vi "Relay_Load_and_PV_v02 (9039).vi"() -> ()   [LabVIEW 2015]
uses:
  subVIs/Load case typedef.ctl
  <vilib>/Modbus/slave/Create Slave Instance (TCP).vi
  <vilib>/FPGAPlugInAG/cRIO-9039/niLvFpga_Open_cRIO-9039.vi
  <vilib>/rvi/interface/common/dynamic/niFpgaDynamicAddResources.vi
  <vilib>/Utility/error.llb/Error Cluster From Error Code.vi
  <vilib>/rvi/errors/niLvFpgaAdjustHostInterfaceError.vi
  <vilib>/FPGAPlugInAG/Dynamic/niLvFpga_Close_Dynamic.vi
  <vilib>/rvi/interface/nirviOpenFPGA/nirviOpenFPGA.xnode
  FPGA Bitfiles/RTDSLoadControl_FPGATarget_9309.lvbitx
  <vilib>/rvi/interface/nirviReadWriteControl/nirviReadWriteControl.xnode
  <vilib>/rvi/interface/nirviCloseFPGA/nirviCloseFPGA.xnode
  <vilib>/Modbus/slave/Modbus Slave.lvclass
  2015 SP1 Support Files/Project Dependencies/Common/Modbus Data Conversion.llb/Modbus Data Conversion.lvlib
  NiFpgaLv.dll
  <vilib>/rvi/interface/Simulation/niFpgaSimulationCallBeginRW.vi
panel:
  out "error out":errorcluster
  out "Load array":sgl[](array[numeric])
  out "PV array":sgl[](array[numeric])
  out "Loop dT (Ticks)":u32
  in  "Loop Rate (Ticks)":u32=1000
  out "Activate Command PV":bool
  out "Deactivate Command PV":bool
  out "Activation Status PV":bool
  out "Deactivation Status PV":bool=TRUE
  out "TCP \nConnection Count PV":u32
  out "comm stopped PV":bool
  in  "Input register\naddresses PV":T1={"Ia"=30030, "Ib"=30040, "Ic"=30050, "Va"=30130, "Vb"=30140, "Vc"=30150, "Pa"=30230, "Pb"=30240, "Pc"=30250, "Qa"=30330, "Qb"=30340, "Qc"=30350}
  in  "Input \nregister values PV":T2
  out "Modbus Data PV":T3
  out "S Total PV":dbl
  out "P Total PV":dbl
  out "Q Total PV":dbl
  out "Q Total":dbl
  out "P Total":dbl
  out "S Total":dbl
  out "Modbus Data":T3
  in  "Input \nregister values":T3
  out "comm stopped":bool
  out "Activate Command":bool
  out "Deactivate Command":bool
  out "Activation Status":bool
  out "Deactivation Status":bool=TRUE
  out "TCP \nConnection Count":u32
  in  "Input register\naddresses":T1={"Ia"=30030, "Ib"=30040, "Ic"=30050, "Va"=30130, "Vb"=30140, "Vc"=30150, "Pa"=30230, "Pb"=30240, "Pc"=30250, "Qa"=30330, "Qb"=30340, "Qc"=30350}
  in  "stop":bool
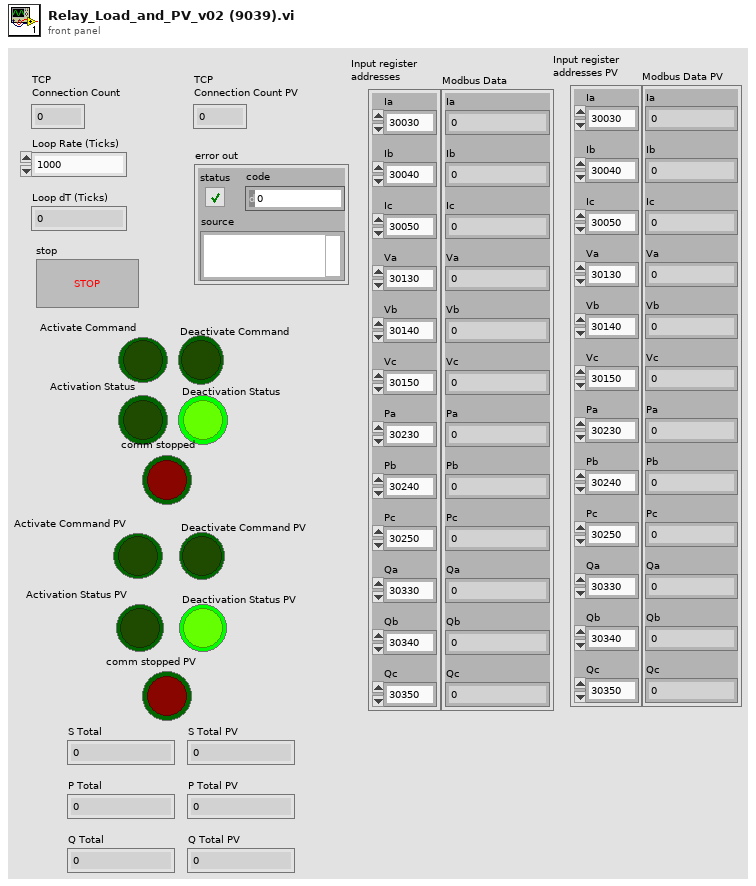
[diagram p1: front panel]
types:
  T1 = cluster{"Ia":u16, "Ib":u16, "Ic":u16, "Va":u16, "Vb":u16, "Vc":u16, "Pa":u16, "Pb":u16, "Pc":u16, "Qa":u16, "Qb":u16, "Qc":u16}
  T2 = cluster{"Ia PV":dbl, "Ib PV":dbl, "Ic PV":dbl, "Va PV":dbl, "Vb PV":dbl, "Vc PV":dbl, "Pa PV":dbl, "Pb PV":dbl, "Pc PV":dbl, "Qa PV":dbl, "Qb PV":dbl, "Qc PV":dbl}
  T3 = cluster{"Ia":dbl, "Ib":dbl, "Ic":dbl, "Va":dbl, "Vb":dbl, "Vc":dbl, "Pa":dbl, "Pb":dbl, "Pc":dbl, "Qa":dbl, "Qb":dbl, "Qc":dbl}
  T4 = typedef "Load case typedef.ctl" = enum16{"Commisioning", "Activation", "Deactivation"}
  T5 = cluster{dbl, dbl, dbl, dbl, dbl, dbl, dbl, dbl, dbl, dbl, dbl, dbl}
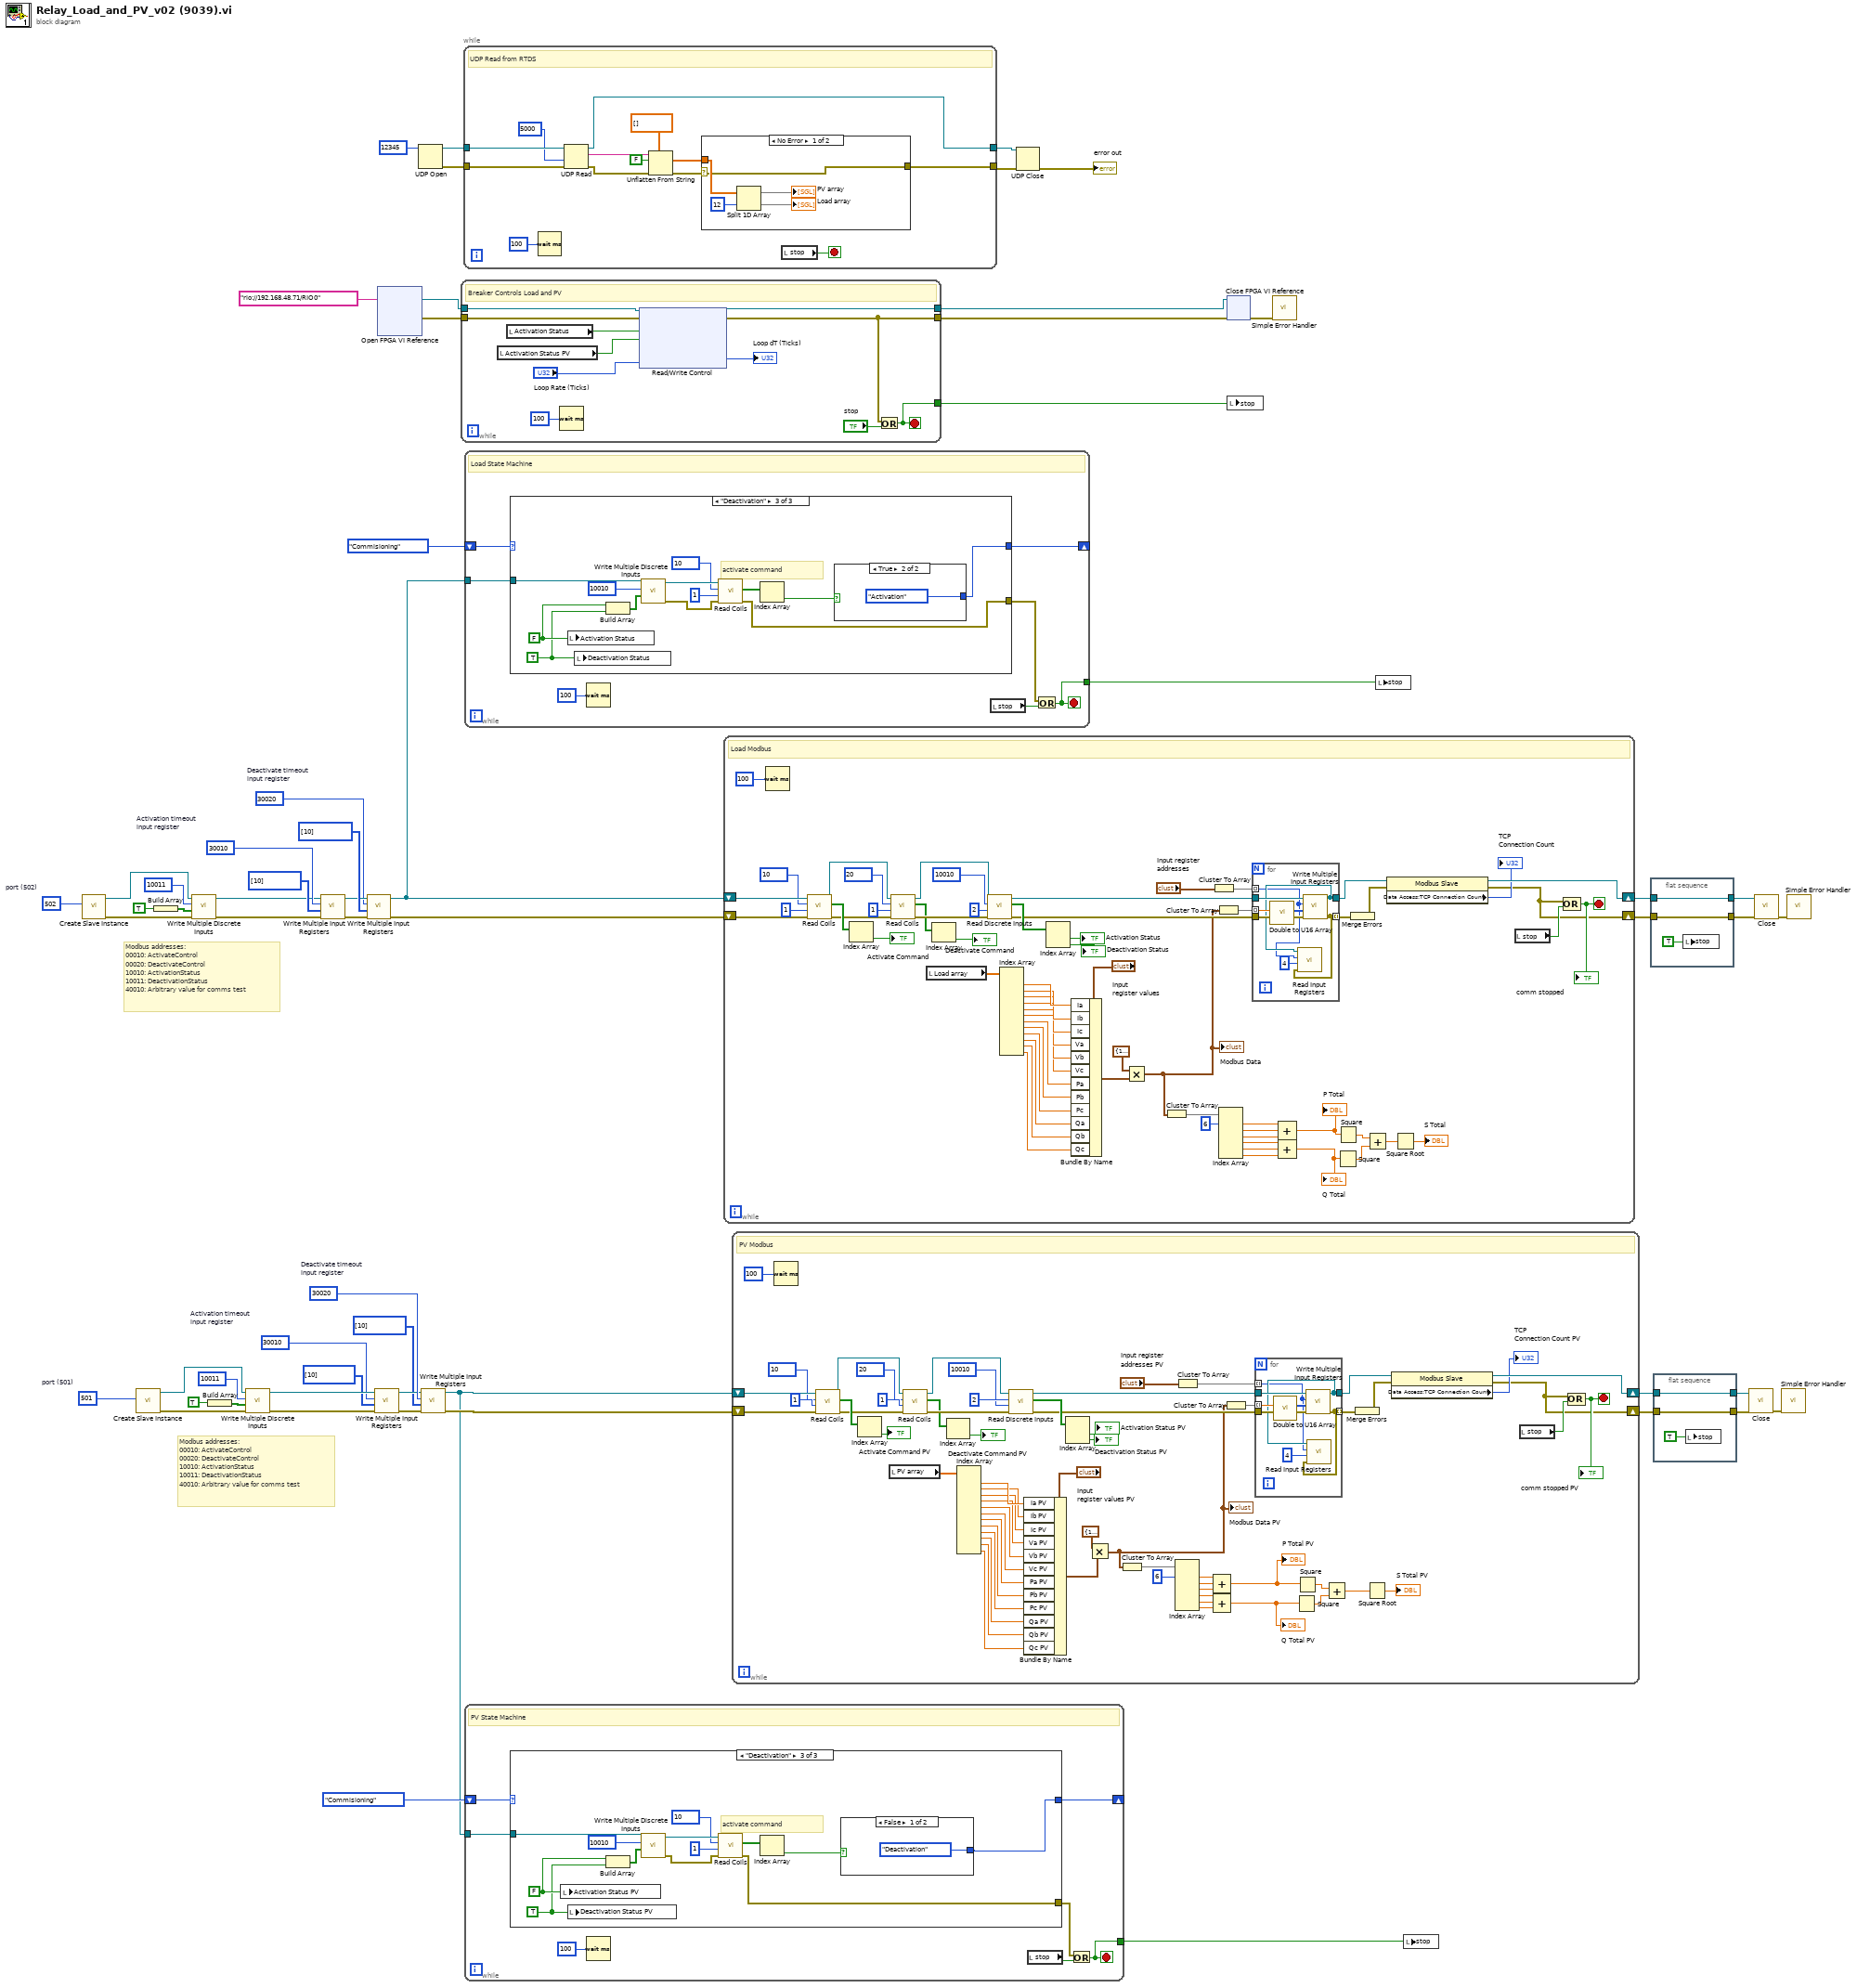
[diagram p0: block diagram]
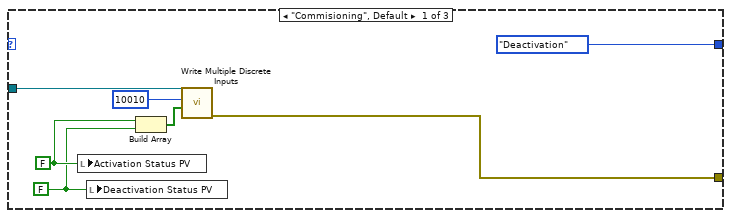
[diagram p3: hidden frame]
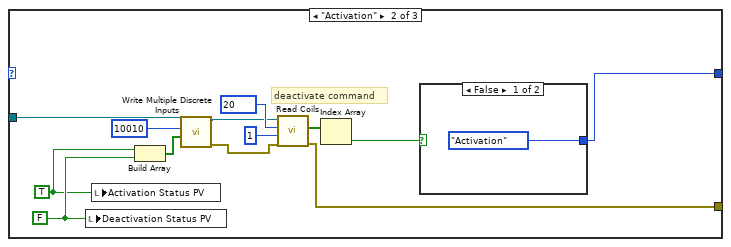
[diagram p4: hidden frame]
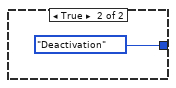
[diagram p5: hidden frame]
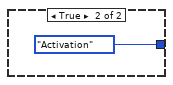
[diagram p6: hidden frame]
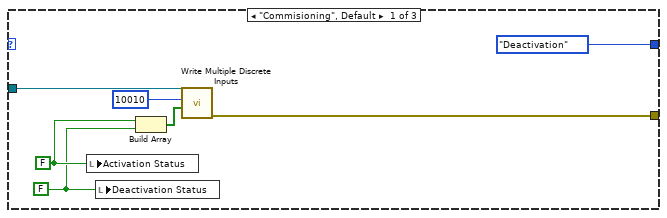
[diagram p7: hidden frame]
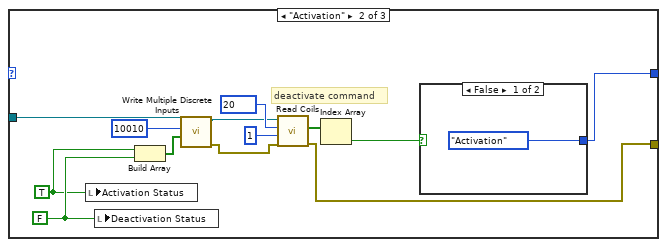
[diagram p8: hidden frame]
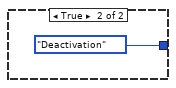
[diagram p9: hidden frame]
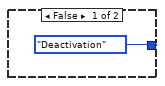
[diagram p10: hidden frame]
diagram:
  w28 = u16 501  # port (501)
  w32 = u16 30020  # Deactivate timeout input register
  w34 = u16 30010  # Activation timeout input register
  w53 = u16 502  # port (502)
  w45 = u16 30020  # Deactivate timeout input register
  w43 = u16 30010  # Activation timeout input register
  # "Modbus addresses:\n00010: ActivateControl\n00020: DeactivateControl\n10010: ActivationStatus\n10011: DeactivationStatus\n40010: Arbitrary value for comms test"
  # "Modbus addresses:\n00010: ActivateControl\n00020: DeactivateControl\n10010: ActivationStatus\n10011: DeactivationStatus\n40010: Arbitrary value for comms test"
  n1 = call-poly <vilib>:"Create Slave Instance.vi"("port (502)"=w53) -> ("error out"=w57:errorcluster, "TCP slave instance"=w58:refnum<class "Modbus Slave.lvclass">)  [unwired: 9 in]
  n2 = call-poly <vilib>:"Create Slave Instance.vi"("port (502)"=w28) -> ("error out"=w24:errorcluster, "TCP slave instance"=w23:refnum<class "Modbus Slave.lvclass">)  [unwired: 9 in]
  n3 = Build Array(TRUE ("Activate 2")) -> (w54:bool[])
  n4 = call-dynamic "Write Multiple Discrete Inputs.vi"("error in (no error)"=w57, "discrete input values"=w54, "starting address"=u16 10011, "Modbus slave in"=w58) -> ("error out"=w41:errorcluster, "Modbus slave out"=w42:refnum<class "Modbus Slave.lvclass">)  [unwired: 6 in]
  n5 = Build Array(TRUE ("Activate 2")) -> (w27:bool[])
  n6 = call-dynamic "Write Multiple Discrete Inputs.vi"("error in (no error)"=w24, "discrete input values"=w27, "starting address"=u16 10011, "Modbus slave in"=w23) -> ("error out"=w36:errorcluster, "Modbus slave out"=w35:refnum<class "Modbus Slave.lvclass">)  [unwired: 6 in]
  n7 = call-dynamic "Write Multiple Input Registers.vi"("error in (no error)"=w41, "input register values"=u16[] [10], "starting address"=w43, "Modbus slave in"=w42) -> ("error out"=w47:errorcluster, "Modbus slave out"=w46:refnum<class "Modbus Slave.lvclass">)  [unwired: 6 in]
  n8 = call-dynamic "Write Multiple Input Registers.vi"("error in (no error)"=w47, "input register values"=u16[] [10], "starting address"=w45, "Modbus slave in"=w46) -> ("error out"=w39:errorcluster, "Modbus slave out"=w40:refnum<class "Modbus Slave.lvclass">)  [unwired: 6 in]
  n9 = call-dynamic "Write Multiple Input Registers.vi"("error in (no error)"=w36, "input register values"=u16[] [10], "starting address"=w34, "Modbus slave in"=w35) -> ("error out"=w30:errorcluster, "Modbus slave out"=w31:refnum<class "Modbus Slave.lvclass">)  [unwired: 6 in]
  n10 = xnode "Open FPGA VI Reference"("resource name"=tag "rio://192.168.48.71/RIO0") -> ("FPGA VI Reference Out"=w51:refnum<k20>, "error out"=w50:errorcluster)  [unwired: 1 in]
  n11 = UDP Open(11:u16 12345 ("port")) -> (port=w4:refnum<k16>, 0:w3:errorcluster)  [unwired: 4 in, 1 out]
  n12 = call-dynamic "Write Multiple Input Registers.vi"("error in (no error)"=w30, "input register values"=u16[] [10], "starting address"=w32, "Modbus slave in"=w31) -> ("error out"=w22:errorcluster, "Modbus slave out"=w19:refnum<class "Modbus Slave.lvclass">)  [unwired: 6 in]
  n13 = while {
    tunnel: [w70] -> w52
    tunnel: w51 -> [w69]
    tunnel: w50 -> [w68]
    tunnel: [w61] -> w49
    tunnel: [w60] -> w9
    stop <- w60 stop-if-true
    # "Breaker Controls Load and PV"
    n14 = local read "Activation Status PV"() -> (w65:bool)
    n15 = local read "Activation Status"() -> (w67:bool)
    n16 = Wait (ms)(milliseconds to wait=u32 100) -> ()  [unwired: 1 out]
    n17 = xnode "Read/Write Control"("FPGA VI Reference In"=w69, "error in"=w68, "Load Relay closed"=w67, "PV Relay closed"=w65, "Loop Rate (Ticks)"="Loop Rate (Ticks)") -> ("FPGA VI Reference Out"=w70:refnum<k20>, "error out"=w61:errorcluster, "Loop dT (Ticks)"=→"Loop dT (Ticks)":u32)
    n18 = Or(x=w61, y="stop") -> (x .or. y?=w60:bool)
  }
  n19 = while {
    tunnel: [w75] -> w2
    tunnel: [w74] -> w5
    tunnel: w4 -> [w73]
    tunnel: w3 -> [w72]
    stop <- w83 stop-if-true
    # "UDP Read from RTDS"
    n20 = Wait (ms)(milliseconds to wait=u32 100) -> ()  [unwired: 1 out]
    n21 = UDP Read(connection ID=w73, timeout ms (25000)=5000, 8:w72) -> (data out=w82:string, error out=w81:errorcluster, 3:w74:refnum<k16>)  [unwired: 1 in, 2 out]
    n22 = Unflatten From String(type=sgl[] [], binary string=w82, data includes array or string size? (T)=FALSE, error in (no error)=w81) -> (value=w78:sgl[], error out=w77:errorcluster)  [unwired: 1 in, 1 out]
    n23 = case shown="No Error" w77 {
      selector: w77 -> [w84 w89]
      tunnel: w78 -> [w88 _]
      tunnel: [w84 w89] -> w75
      frame No Error {
        n24 = Split 1D Array(array=w88, index=12 ("length")) -> (first subarray=→"PV array":sgl[], second subarray=→"Load array":sgl[])
      }
      frame Error {
      }
    }
    n25 = local read "stop"() -> (w83:bool)
  }
  n26 = while {
    tunnel: w40 -> [w94]
    shift-right: [w93] -> _
    shift-left: Load_case_typedef."Commisioning" ("Load enum") -> [w95]
    tunnel: [w90] -> w8
    stop <- w90 stop-if-true
    # "Load State Machine"
    n27 = case shown="\"Deactivation\"" w95 {
      tunnel: w94 -> [w101 w112 w127]
      tunnel: [Load_case_typedef."Deactivation" ("Load enum") w106 w121] -> w93
      tunnel: [w97 w104 w119] -> w92
      frame "Commisioning", Default {
        w99 = FALSE ("Deactivation Status")
        w100 = FALSE ("Activation Status")
        n28 = local write "Activation Status"(w100) -> ()
        n29 = local write "Deactivation Status"(w99) -> ()
        n30 = Build Array(w100, w99) -> (w103:bool[])
        n31 = call-dynamic "Write Multiple Discrete Inputs.vi"("discrete input values"=w103, "starting address"=u16 10010, "Modbus slave in"=w101) -> ("error out"=w97:errorcluster)  [unwired: 7 in, 1 out]
      }
      frame "Activation" {
        w116 = FALSE ("Deactivation Status")
        w115 = TRUE ("Activation Status")
        # "deactivate command"
        n32 = local write "Activation Status"(w115) -> ()
        n33 = local write "Deactivation Status"(w116) -> ()
        n34 = Build Array(w115, w116) -> (w113:bool[])
        n35 = call-dynamic "Write Multiple Discrete Inputs.vi"("discrete input values"=w113, "starting address"=u16 10010, "Modbus slave in"=w112) -> ("error out"=w105:errorcluster, "Modbus slave out"=w108:refnum<class "Modbus Slave.lvclass">)  [unwired: 7 in]
        n36 = call-dynamic "Read Coils.vi"("error in (no error)"=w105, "number of coils"=u16 1, "starting address"=u16 20, "Modbus slave in"=w108) -> ("error out"=w104:errorcluster, "coil values"=w109:bool[])  [unwired: 5 in, 1 out]
        n37 = Index Array(array=w109) -> (element=w107:bool)  [unwired: 1 in]
        n38 = case shown="False" w107 {
          tunnel: [Load_case_typedef."Activation" ("Load enum") Load_case_typedef."Deactivation" ("Load enum")] -> w106
          frame False {
          }
          frame True {
          }
        }
      }
      frame "Deactivation" {
        w128 = TRUE ("Deactivation Status")
        w129 = FALSE ("Activation Status")
        # "activate command"
        n39 = local write "Activation Status"(w129) -> ()
        n40 = local write "Deactivation Status"(w128) -> ()
        n41 = Build Array(w129, w128) -> (w131:bool[])
        n42 = call-dynamic "Write Multiple Discrete Inputs.vi"("discrete input values"=w131, "starting address"=u16 10010, "Modbus slave in"=w127) -> ("error out"=w120:errorcluster, "Modbus slave out"=w126:refnum<class "Modbus Slave.lvclass">)  [unwired: 7 in]
        n43 = call-dynamic "Read Coils.vi"("error in (no error)"=w120, "number of coils"=u16 1, "starting address"=u16 10, "Modbus slave in"=w126) -> ("error out"=w119:errorcluster, "coil values"=w123:bool[])  [unwired: 5 in, 1 out]
        n44 = Index Array(array=w123) -> (element=w122:bool)  [unwired: 1 in]
        n45 = case shown="True" w122 {
          tunnel: [Load_case_typedef."Deactivation" ("Load enum") Load_case_typedef."Activation" ("Load enum")] -> w121
          frame False {
          }
          frame True {
          }
        }
      }
    }
    n46 = Wait (ms)(milliseconds to wait=u32 100) -> ()  [unwired: 1 out]
    n47 = local read "stop"() -> (w91:bool)
    n48 = Or(x=w92, y=w91) -> (x .or. y?=w90:bool)
  }
  n49 = while {
    tunnel: w19 -> [w138]
    shift-right: [w137] -> _
    shift-left: Load_case_typedef."Commisioning" ("Load enum") -> [w139]
    tunnel: [w134] -> w7
    stop <- w134 stop-if-true
    # "PV State Machine"
    n50 = case shown="\"Deactivation\"" w139 {
      tunnel: w138 -> [w145 w156 w171]
      tunnel: [Load_case_typedef."Deactivation" ("Load enum") w150 w165] -> w137
      tunnel: [w141 w148 w163] -> w135
      frame "Commisioning", Default {
        w143 = FALSE ("Deactivation Status")
        w144 = FALSE ("Activation Status")
        n51 = local write "Activation Status PV"(w144) -> ()
        n52 = local write "Deactivation Status PV"(w143) -> ()
        n53 = Build Array(w144, w143) -> (w147:bool[])
        n54 = call-dynamic "Write Multiple Discrete Inputs.vi"("discrete input values"=w147, "starting address"=u16 10010, "Modbus slave in"=w145) -> ("error out"=w141:errorcluster)  [unwired: 7 in, 1 out]
      }
      frame "Activation" {
        w160 = FALSE ("Deactivation Status")
        w159 = TRUE ("Activation Status")
        # "deactivate command"
        n55 = local write "Deactivation Status PV"(w160) -> ()
        n56 = local write "Activation Status PV"(w159) -> ()
        n57 = Build Array(w159, w160) -> (w157:bool[])
        n58 = call-dynamic "Write Multiple Discrete Inputs.vi"("discrete input values"=w157, "starting address"=u16 10010, "Modbus slave in"=w156) -> ("error out"=w149:errorcluster, "Modbus slave out"=w152:refnum<class "Modbus Slave.lvclass">)  [unwired: 7 in]
        n59 = call-dynamic "Read Coils.vi"("error in (no error)"=w149, "number of coils"=u16 1, "starting address"=u16 20, "Modbus slave in"=w152) -> ("error out"=w148:errorcluster, "coil values"=w153:bool[])  [unwired: 5 in, 1 out]
        n60 = Index Array(array=w153) -> (element=w151:bool)  [unwired: 1 in]
        n61 = case shown="False" w151 {
          tunnel: [Load_case_typedef."Activation" ("Load enum") Load_case_typedef."Deactivation" ("Load enum")] -> w150
          frame False {
          }
          frame True {
          }
        }
      }
      frame "Deactivation" {
        w172 = TRUE ("Deactivation Status")
        w173 = FALSE ("Activation Status")
        # "activate command"
        n62 = local write "Activation Status PV"(w173) -> ()
        n63 = local write "Deactivation Status PV"(w172) -> ()
        n64 = Build Array(w173, w172) -> (w175:bool[])
        n65 = call-dynamic "Write Multiple Discrete Inputs.vi"("discrete input values"=w175, "starting address"=u16 10010, "Modbus slave in"=w171) -> ("error out"=w164:errorcluster, "Modbus slave out"=w170:refnum<class "Modbus Slave.lvclass">)  [unwired: 7 in]
        n66 = call-dynamic "Read Coils.vi"("error in (no error)"=w164, "number of coils"=u16 1, "starting address"=u16 10, "Modbus slave in"=w170) -> ("error out"=w163:errorcluster, "coil values"=w167:bool[])  [unwired: 5 in, 1 out]
        n67 = Index Array(array=w167) -> (element=w166:bool)  [unwired: 1 in]
        n68 = case shown="False" w166 {
          tunnel: [Load_case_typedef."Deactivation" ("Load enum") Load_case_typedef."Activation" ("Load enum")] -> w165
          frame False {
          }
          frame True {
          }
        }
      }
    }
    n69 = Wait (ms)(milliseconds to wait=u32 100) -> ()  [unwired: 1 out]
    n70 = local read "stop"() -> (w136:bool)
    n71 = Or(x=w135, y=w136) -> (x .or. y?=w134:bool)
  }
  n72 = while {
    shift-right: [w221] -> w16
    shift-left: w40 -> [w237]
    shift-right: [w178] -> w17
    shift-left: w39 -> [w236]
    stop <- w240 stop-if-true
    # "Load Modbus"
    n73 = Wait (ms)(milliseconds to wait=u32 100) -> ()  [unwired: 1 out]
    n74 = call-dynamic "Read Coils.vi"("error in (no error)"=w236, "number of coils"=u16 1, "starting address"=u16 10, "Modbus slave in"=w237) -> ("error out"=w229:errorcluster, "coil values"=w241:bool[], "Modbus slave out"=w226:refnum<class "Modbus Slave.lvclass">)  [unwired: 5 in]
    n75 = Index Array(array=w241) -> (element=→"Activate Command":bool)  [unwired: 1 in]
    n76 = call-dynamic "Read Coils.vi"("error in (no error)"=w229, "number of coils"=u16 1, "starting address"=u16 20, "Modbus slave in"=w226) -> ("error out"=w228:errorcluster, "coil values"=w223:bool[], "Modbus slave out"=w227:refnum<class "Modbus Slave.lvclass">)  [unwired: 5 in]
    n77 = local read "Load array"() -> (w194:sgl[])
    n78 = Index Array(array=w223) -> (element=→"Deactivate Command":bool)  [unwired: 1 in]
    n79 = call-dynamic "Read Discrete Inputs.vi"("error in (no error)"=w228, "number of discrete inputs"=u16 2 ("number of coils"), "starting address"=u16 10010 ("address"), "Modbus slave in"=w227) -> ("error out"=w218:errorcluster, "discrete input values"=w234:bool[], "Modbus slave out"=w219:refnum<class "Modbus Slave.lvclass">)  [unwired: 5 in]
    n80 = Index Array(array=w194) -> (element #1=w193:sgl, element #2=w192:sgl, element #3=w191:sgl, element #4=w190:sgl, element #5=w189:sgl, element #6=w188:sgl, element #7=w187:sgl, element #8=w186:sgl, element #9=w185:sgl, element #10=w184:sgl, element #11=w183:sgl, element #12=w182:sgl)  [unwired: 12 in]
    n81 = Index Array(array=w234) -> (element #1=→"Activation Status":bool, element #2=→"Deactivation Status":bool)  [unwired: 2 in]
    n82 = Bundle By Name(cluster="Input \nregister values", "Ia"=w193, "Ib"=w192, "Ic"=w191, "Va"=w190, "Vb"=w189, "Vc"=w188, "Pa"=w187, "Pb"=w186, "Pc"=w185, "Qa"=w184, "Qb"=w183, "Qc"=w182) -> (w215:T3)
    n83 = Multiply(x=T3 {"Ia"=1000.0, "Ib"=1000.0, "Ic"=1000.0, "Va"=1732.0, "Vb"=1732.0, "Vc"=1732.0, "Pa"=1000000.0, "Pb"=1000000.0, "Pc"=1000000.0, "Qa"=1000000.0, "Qb"=1000000.0, "Qc"=1000000.0}, y=w215) -> (x*y=w180:T3)
    "Modbus Data" <- w180
    n84 = Cluster To Array(cluster=w180) -> (array=w181:dbl[])
    n85 = Cluster To Array(cluster="Input register\naddresses") -> (array=w206:u16[])
    n86 = Cluster To Array(cluster=w180) -> (array=w205:dbl[])
    n87 = Index Array(array=w181, index #1=6 ("index")) -> (element #1=w200:dbl, element #2=w199:dbl, element #3=w198:dbl, element #4=w197:dbl, element #5=w195:dbl, element #6=w196:dbl)  [unwired: 5 in]
    n88 = for {
      tunnel: w219 -> [w249]
      tunnel: w218 -> [w248]
      tunnel: [w245] -> w204
      tunnel: [w242] -> w208 mode=indexing
      tunnel: w206 -> [w244] mode=indexing
      tunnel: w205 -> [w246] mode=indexing
      n89 = call "Double to U16 Array.vi"("Double"=w246) -> ("U16 Array"=w247:u16[])  [unwired: 10 in]
      n90 = call-dynamic "Write Multiple Input Registers.vi"("error in (no error)"=w248, "input register values"=w247, "starting address"=w244, "Modbus slave in"=w249) -> ("error out"=w242:errorcluster, "Modbus slave out"=w245:refnum<class "Modbus Slave.lvclass">)  [unwired: 6 in]
      n91 = call-dynamic "Read Input Registers.vi"("error in (no error)"=w242, "number of input registers"=u16 4 ("number of coils"), "starting address"=w244, "Modbus slave in"=w245) -> ()  [unwired: 5 in, 3 out]
    }
    n92 = Compound Arithmetic op=ADD(w200, w199, w198) -> (w201:dbl)
    "P Total" <- w201
    n93 = Compound Arithmetic op=ADD(w197, w195, w196) -> (w202:dbl)
    "Q Total" <- w202
    n94 = Square(x=w202) -> (x^2=w212:dbl)
    n95 = Square(x=w201) -> (x^2=w213:dbl)
    n96 = Merge Errors(w208) -> (w179:errorcluster)
    n97 = Add(x=w213, y=w212) -> (x+y=w211:dbl)
    n98 = property class="Modbus Slave"(reference=w204, error in=w179) -> (reference out=w221:refnum<class "Modbus Slave.lvclass">, error out=w178:errorcluster, "Data Access:TCP Connection Count"=→"TCP \nConnection Count":u32)
    n99 = Square Root(x=w211) -> (sqrt(x)=→"S Total":dbl)
    n100 = local read "stop"() -> (w214:bool)
    n101 = Compound Arithmetic op=OR(w178, w214) -> (w240:bool)
    "comm stopped" <- w240
  }
  n102 = while {
    shift-right: [w293] -> w13
    shift-left: w19 -> [w309]
    shift-right: [w250] -> w12
    shift-left: w22 -> [w308]
    stop <- w312 stop-if-true
    # "PV Modbus"
    n103 = Wait (ms)(milliseconds to wait=u32 100) -> ()  [unwired: 1 out]
    n104 = call-dynamic "Read Coils.vi"("error in (no error)"=w308, "number of coils"=u16 1, "starting address"=u16 10, "Modbus slave in"=w309) -> ("error out"=w301:errorcluster, "coil values"=w313:bool[], "Modbus slave out"=w298:refnum<class "Modbus Slave.lvclass">)  [unwired: 5 in]
    n105 = Index Array(array=w313) -> (element=→"Activate Command PV":bool)  [unwired: 1 in]
    n106 = local read "PV array"() -> (w272:sgl[])
    n107 = call-dynamic "Read Coils.vi"("error in (no error)"=w301, "number of coils"=u16 1, "starting address"=u16 20, "Modbus slave in"=w298) -> ("error out"=w300:errorcluster, "coil values"=w295:bool[], "Modbus slave out"=w299:refnum<class "Modbus Slave.lvclass">)  [unwired: 5 in]
    n108 = Index Array(array=w295) -> (element=→"Deactivate Command PV":bool)  [unwired: 1 in]
    n109 = Index Array(array=w272) -> (element #1=w271:sgl, element #2=w270:sgl, element #3=w269:sgl, element #4=w268:sgl, element #5=w267:sgl, element #6=w266:sgl, element #7=w265:sgl, element #8=w264:sgl, element #9=w263:sgl, element #10=w262:sgl, element #11=w261:sgl, element #12=w260:sgl)  [unwired: 12 in]
    n110 = call-dynamic "Read Discrete Inputs.vi"("error in (no error)"=w300, "number of discrete inputs"=u16 2 ("number of coils"), "starting address"=u16 10010 ("address"), "Modbus slave in"=w299) -> ("error out"=w274:errorcluster, "discrete input values"=w306:bool[], "Modbus slave out"=w275:refnum<class "Modbus Slave.lvclass">)  [unwired: 5 in]
    n111 = Bundle By Name(cluster="Input \nregister values PV", "Ia PV"=w271, "Ib PV"=w270, "Ic PV"=w269, "Va PV"=w268, "Vb PV"=w267, "Vc PV"=w266, "Pa PV"=w265, "Pb PV"=w264, "Pc PV"=w263, "Qa PV"=w262, "Qb PV"=w261, "Qc PV"=w260) -> (w282:T2)
    n112 = Index Array(array=w306) -> (element #1=→"Activation Status PV":bool, element #2=→"Deactivation Status PV":bool)  [unwired: 2 in]
    n113 = Multiply(x=T3 {"Ia"=1000.0, "Ib"=1000.0, "Ic"=1000.0, "Va"=1732.0, "Vb"=1732.0, "Vc"=1732.0, "Pa"=1000000.0, "Pb"=1000000.0, "Pc"=1000000.0, "Qa"=1000000.0, "Qb"=1000000.0, "Qc"=1000000.0}, y=w282) -> (x*y=w252:T5)
    "Modbus Data PV" <- w252
    n114 = Cluster To Array(cluster=w252) -> (array=w259:dbl[])
    n115 = Index Array(array=w259, index #1=6 ("index")) -> (element #1=w258:dbl, element #2=w257:dbl, element #3=w256:dbl, element #4=w255:dbl, element #5=w254:dbl, element #6=w253:dbl)  [unwired: 5 in]
    n116 = Cluster To Array(cluster="Input register\naddresses PV") -> (array=w278:u16[])
    n117 = Compound Arithmetic op=ADD(w258, w257, w256) -> (w288:dbl)
    "P Total PV" <- w288
    n118 = Compound Arithmetic op=ADD(w255, w254, w253) -> (w283:dbl)
    "Q Total PV" <- w283
    n119 = Cluster To Array(cluster=w252) -> (array=w289:dbl[])
    n120 = for {
      tunnel: w275 -> [w321]
      tunnel: w274 -> [w320]
      tunnel: [w316] -> w276
      tunnel: [w314] -> w277 mode=indexing
      tunnel: w278 -> [w315] mode=indexing
      tunnel: w289 -> [w318] mode=indexing
      n121 = call "Double to U16 Array.vi"("Double"=w318) -> ("U16 Array"=w319:u16[])  [unwired: 10 in]
      n122 = call-dynamic "Write Multiple Input Registers.vi"("error in (no error)"=w320, "input register values"=w319, "starting address"=w315, "Modbus slave in"=w321) -> ("error out"=w314:errorcluster, "Modbus slave out"=w316:refnum<class "Modbus Slave.lvclass">)  [unwired: 6 in]
      n123 = call-dynamic "Read Input Registers.vi"("error in (no error)"=w314, "number of input registers"=u16 4 ("number of coils"), "starting address"=w315, "Modbus slave in"=w316) -> ()  [unwired: 5 in, 3 out]
    }
    n124 = Square(x=w283) -> (x^2=w285:dbl)
    n125 = Square(x=w288) -> (x^2=w284:dbl)
    n126 = Add(x=w284, y=w285) -> (x+y=w286:dbl)
    n127 = Merge Errors(w277) -> (w251:errorcluster)
    n128 = Square Root(x=w286) -> (sqrt(x)=→"S Total PV":dbl)
    n129 = property class="Modbus Slave"(reference=w276, error in=w251) -> (reference out=w293:refnum<class "Modbus Slave.lvclass">, error out=w250:errorcluster, "Data Access:TCP Connection Count"=→"TCP \nConnection Count PV":u32)
    n130 = local read "stop"() -> (w291:bool)
    n131 = Compound Arithmetic op=OR(w250, w291) -> (w312:bool)
    "comm stopped PV" <- w312
  }
  n132 = UDP Close(connection ID=w5, 8:w2) -> (error out=→"error out":errorcluster)  [unwired: 1 out]
  n133 = xnode "Close FPGA VI Reference"("FPGA VI Reference In"=w52, "error in"=w49) -> ("error out"=w18:errorcluster)
  n134 = local write "stop"(w9) -> ()
  n135 = call <vilib>:"Simple Error Handler.vi"("error in (no error)"=w18) -> ()  [unwired: 4 in, 5 out]
  n136 = local write "stop"(w8) -> ()
  n137 = local write "stop"(w7) -> ()
  n138 = flat-sequence {
    tunnel: w17 -> [w323]
    tunnel: w16 -> [w322]
    tunnel: [w323] -> w15
    tunnel: [w322] -> w14
    frame #0 {
      n139 = local write "stop"(TRUE ("stop")) -> ()
    }
  }
  n140 = flat-sequence {
    tunnel: w12 -> [w326]
    tunnel: w13 -> [w325]
    tunnel: [w326] -> w11
    tunnel: [w325] -> w10
    frame #0 {
      n141 = local write "stop"(TRUE ("stop")) -> ()
    }
  }
  n142 = call-dynamic "Close.vi"("error in (no error)"=w11, "Modbus slave in"=w10) -> ("error out"=w21:errorcluster)  [unwired: 9 in]
  n143 = call-dynamic "Close.vi"("error in (no error)"=w15, "Modbus slave in"=w14) -> ("error out"=w59:errorcluster)  [unwired: 9 in]
  n144 = call <vilib>:"Simple Error Handler.vi"("error in (no error)"=w21) -> ()  [unwired: 4 in, 5 out]
  n145 = call <vilib>:"Simple Error Handler.vi"("error in (no error)"=w59) -> ()  [unwired: 4 in, 5 out]
